vi "Get Number of Wheels.vi"(8 "error in (no error)":errorcluster, 11 "steering frame in":refnum<class "NI_Robotics_Steering Frame.lvclass">) -> (0 "error out":errorcluster, 2 "number of wheels":i32, 3 "steering frame out":refnum<class "NI_Robotics_Steering Frame.lvclass">)   [LabVIEW 2017, in "NI_Robotics_Steering Frame.lvclass"]
uses:
  <vilib>/robotics/Steering/Steering Frame/NI_Robotics_Steering Frame.lvclass
  <vilib>/robotics/Steering/Steering Frame/NI_Robotics_Steering Frame.lvclass/NI_Robotics_Steering Frame.ctl
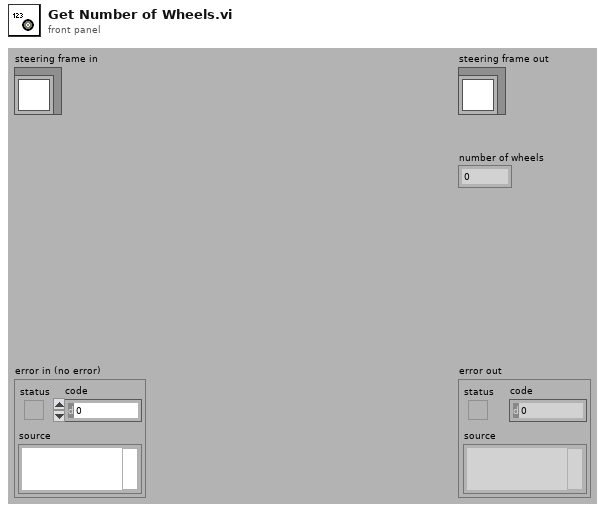
[diagram p1: front panel]
types:
  T1 = typedef "NI_Robotics_Steering Frame.lvclass/Wheel Orientation.ctl" = cluster{"wheel":refnum<class "NI_Robotics_Wheel.lvclass">, "x position":dbl, "y position":dbl, "frame angle (rad)":dbl}
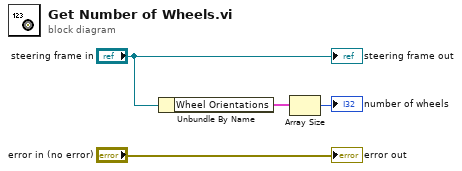
[diagram p0: block diagram]
diagram:
  n1 = Unbundle By Name("steering frame in") -> ("Wheel Orientations"=w2:T1[])
  n2 = Array Size(array=w2) -> (size(s)=→"number of wheels":i32)
  "error out" <- "error in (no error)"
  "steering frame out" <- "steering frame in"
